vi "GetFrameRate.vi"(8 "error in (no error)":errorcluster, 11 "CameraTestingProxyAPI in":refnum<class "CameraTestingProxyAPI.lvclass">) -> (0 "error out":errorcluster, 2 "Frame Rate":u8, 3 "CameraTestingProxyAPI out":refnum<class "CameraTestingProxyAPI.lvclass">)   [LabVIEW 2020, in "CameraTestingProxy.lvlib" / "CameraTestingProxyAPI.lvclass"]
uses:
  CameraTestingProxyAPI.lvclass
  CameraTestingProxyAPI.lvclass/CameraTestingProxyAPI.ctl
  58098f3e-19b0-488c-b3c7-503379fca333.vi
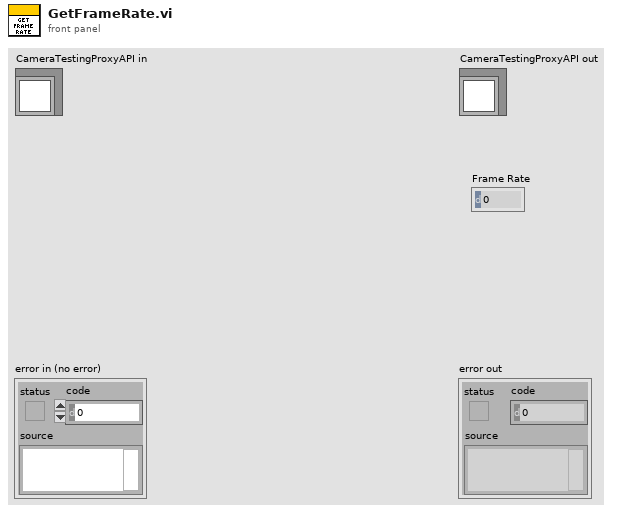
[diagram p1: front panel]
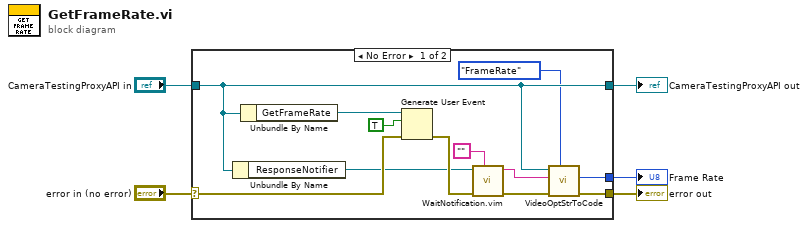
[diagram p0: block diagram]
diagram:
  n1 = case shown="No Error" "error in (no error)" {
    selector: "error in (no error)" -> [w16 w19]
    tunnel: [w8 w19] -> w2
    tunnel: [w9 w18] -> w5
    tunnel: "CameraTestingProxyAPI in" -> [w9 w18]
    tunnel: [w7 _] -> w1
    frame No Error {
      n2 = Unbundle By Name(w9) -> ("ResponseNotifier"=w13:refnum<notifier>)
      n3 = Unbundle By Name(w9) -> ("GetFrameRate"=w17:refnum<user-event>)
      n4 = Generate User Event(user event=w17, event data cluster=TRUE ("event data"), error in=w16) -> (error out=w14:errorcluster)  [unwired: 1 in, 1 out]
      n5 = call "WaitNotification.vim"("Type"="", "error in (no error)"=w14, "ResponseNotifier"=w13) -> ("error out"=w11:errorcluster, "Data"=w10:string)  [unwired: 7 in]
      n6 = call "VideoOptStrToCode.vi"("VideoOption"=enum16{"FrameRate", "ImageType", "Resolution"}."FrameRate", "error in (no error)"=w11, "DescriptionString"=w10, "CameraTestingProxyAPI in"=w9) -> ("error out"=w8:errorcluster, "Code"=w7:u8)  [unwired: 5 in, 1 out]
    }
    frame Error {
    }
  }
  "error out" <- w2
  "CameraTestingProxyAPI out" <- w5
  "Frame Rate" <- w1
